vi "Index_Logic.vi"(0 "X":bool, 4 "Intake Pressed":bool, 6 "B":bool, 7 "Right Trigger":dbl, 8 "Y":bool, 9 "A":bool, 10 "Reject Pressed":bool, 11 "Elevate Pressed":bool) -> ()   [LabVIEW 2020]
uses:
  <vilib>/Rock Robotics/WPI/ThirdParty/Phoenix-LabVIEW/Motor Controller/Controls/CTRE_Phoenix_MotorControl_ControlMode.ctl
  <vilib>/Rock Robotics/WPI/Solenoid/WPI_SolenoidValue.ctl
  <vilib>/Rock Robotics/Network Tables/NT Read String.vi
  <vilib>/Rock Robotics/Network Tables/NT Write Boolean.vi
  <vilib>/Rock Robotics/Network Tables/NT Write Number.vi
  <vilib>/Rock Robotics/WPI/Solenoid/WPI_SolenoidSetEnum.vi
panel:
  in  "Intake want":dbl=0.75
  in  "Elevate want":dbl=-0.35
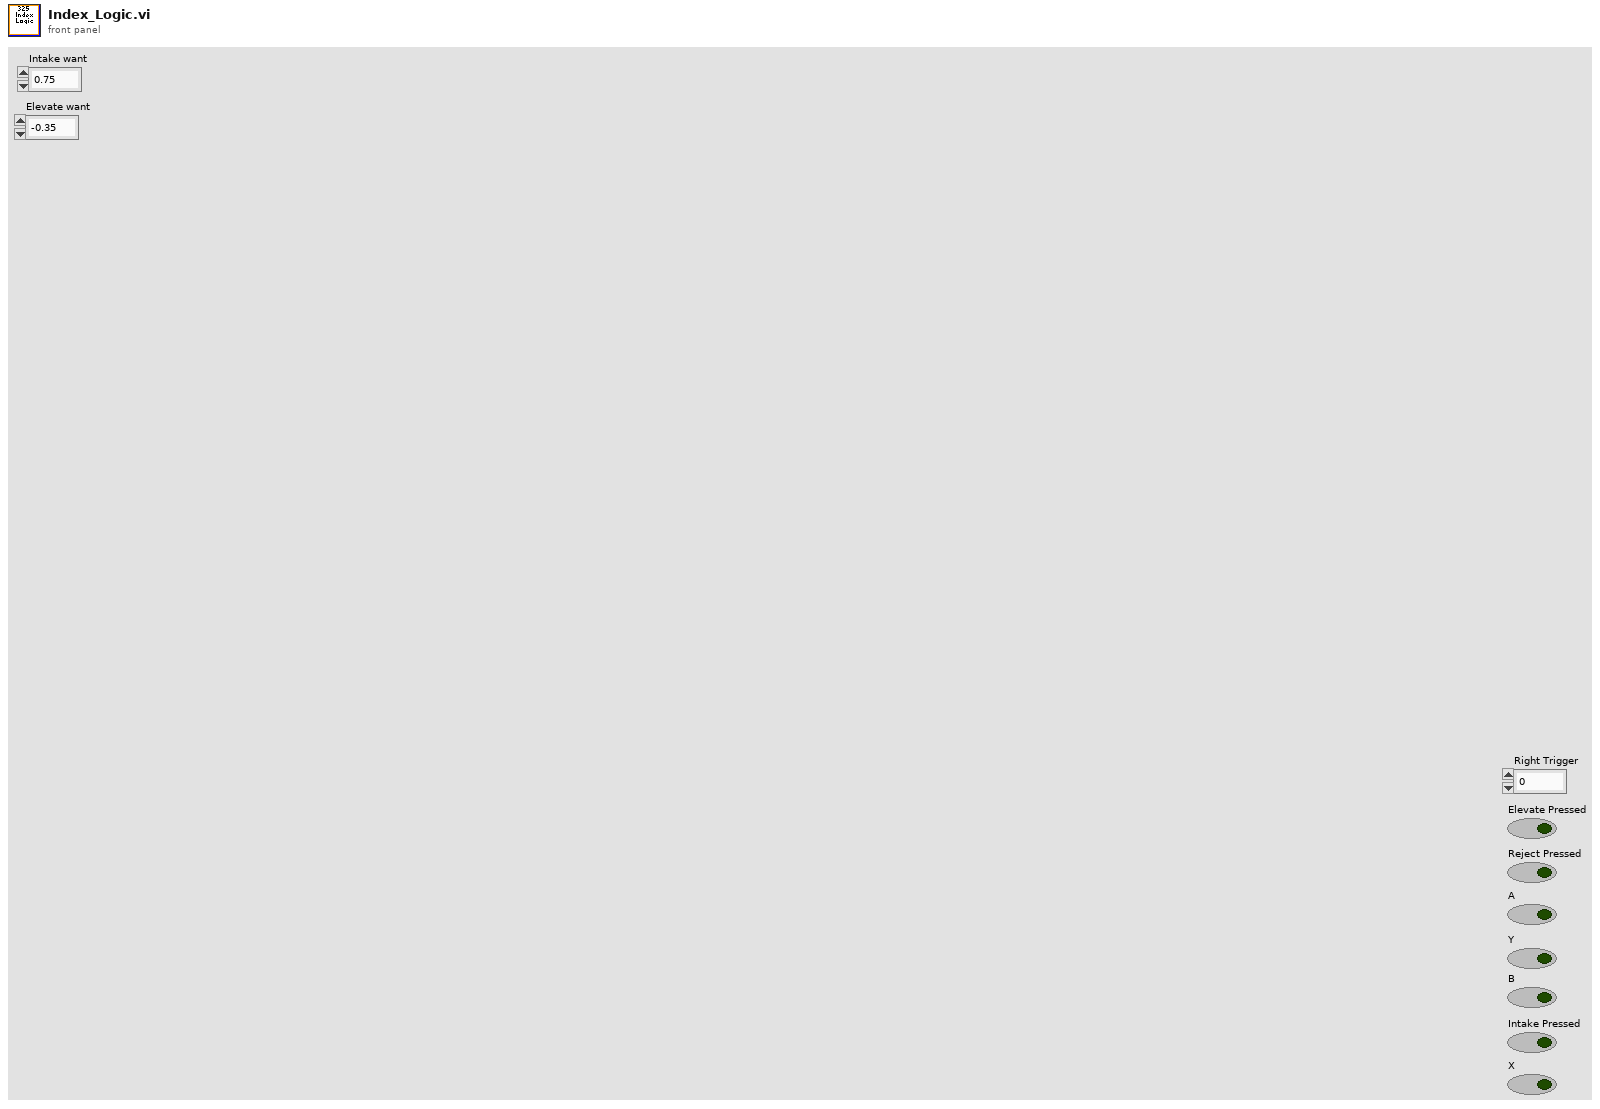
[diagram p1: front panel]
types:
  T1 = typedef "CTRE_Phoenix_MotorControl_ControlMode.ctl" = u16
  T2 = typedef "WPI_SolenoidValue.ctl" = enum16{"Off", "On", "Forward", "Reverse"}
  T3 = typedef "WPI_MotorControlDeviceRef.ctl" = cluster{"DeviceStatus":errorcluster, "Type":T4, "PWM":cluster{"PWM Channel":T5, "DeadBand":T6}, "CAN":cluster{"Device Number":u8, "SetOutput VI Ref":variant, "GetOutput VI Ref":variant, "Enable VI Ref":variant, "Disable VI Ref":variant, "Data":variant}, "Invert":bool, "DIO PWM":cluster{"PWM \"Enable\" Channel":T5, "DIOChannel":T7, "PWM Rate":dbl}}
  T4 = typedef "WPI_MotorControlType.ctl" = enum16{"PWM", "CAN", "DIO PWM"}
  T5 = typedef "FPGA_DIOPWMChannel.ctl" = enum8{"PWM 0", "PWM 1", "PWM 2", "PWM 3", "PWM 4", "PWM 5", "PWM 6", "PWM 7", "PWM 8", "PWM 9", "PWM MXP 0", "PWM MXP 1", "PWM MXP 2", "PWM MXP 3", "PWM MXP 4", "PWM MXP 5", "PWM MXP 6", "PWM MXP 7", "PWM MXP 8", "PWM MXP 9", "Invalid"}
  T6 = typedef "WPI_PWMDeadband.ctl" = cluster{"Name":string, "maxPositivePwm":i32, "minPositivePwm":i32, "centerPwm":i32, "maxNegativePwm":i32, "minNegativePwm":i32, "angularRange":u16}
  T7 = typedef "FPGA_DIOChannel.ctl" = enum8{"DIO 0", "DIO 1", "DIO 2", "DIO 3", "DIO 4", "DIO 5", "DIO 6", "DIO 7", "DIO 8", "DIO 9", "DIO MXP 0", "DIO MXP 1", "DIO MXP 2", "DIO MXP 3", "DIO MXP 4", "DIO MXP 5", "DIO MXP 6", "DIO MXP 7", "DIO MXP 8", "DIO MXP 9", "DIO MXP 10", "DIO MXP 11", "DIO MXP 12", "DIO MXP 13", "DIO MXP 14", "DIO MXP 15", "SPI Port CS1", "SPI Port CS2", "SPI Port CS3", "SPI Port MISO", "SPI Port MOSI", "Invalid"}
  T8 = typedef "WPI_SolenoidDevRef.ctl" = cluster{"DevStatus":errorcluster, "Pneumatics Control Module":u8, "Forward Solenoid Channel":T9, "Reverse Solenoid Channel":T9}
  T9 = typedef "WPI_SolenoidChannel.ctl" = enum8{"Solenoid 0", "Solenoid 1", "Solenoid 2", "Solenoid 3", "Solenoid 4", "Solenoid 5", "Solenoid 6", "Solenoid 7", "Solenoid 8", "Solenoid 9", "Solenoid 10", "Solenoid 11", "Solenoid 12", "Solenoid 13", "Solenoid 14", "Solenoid 15", "Invalid"}
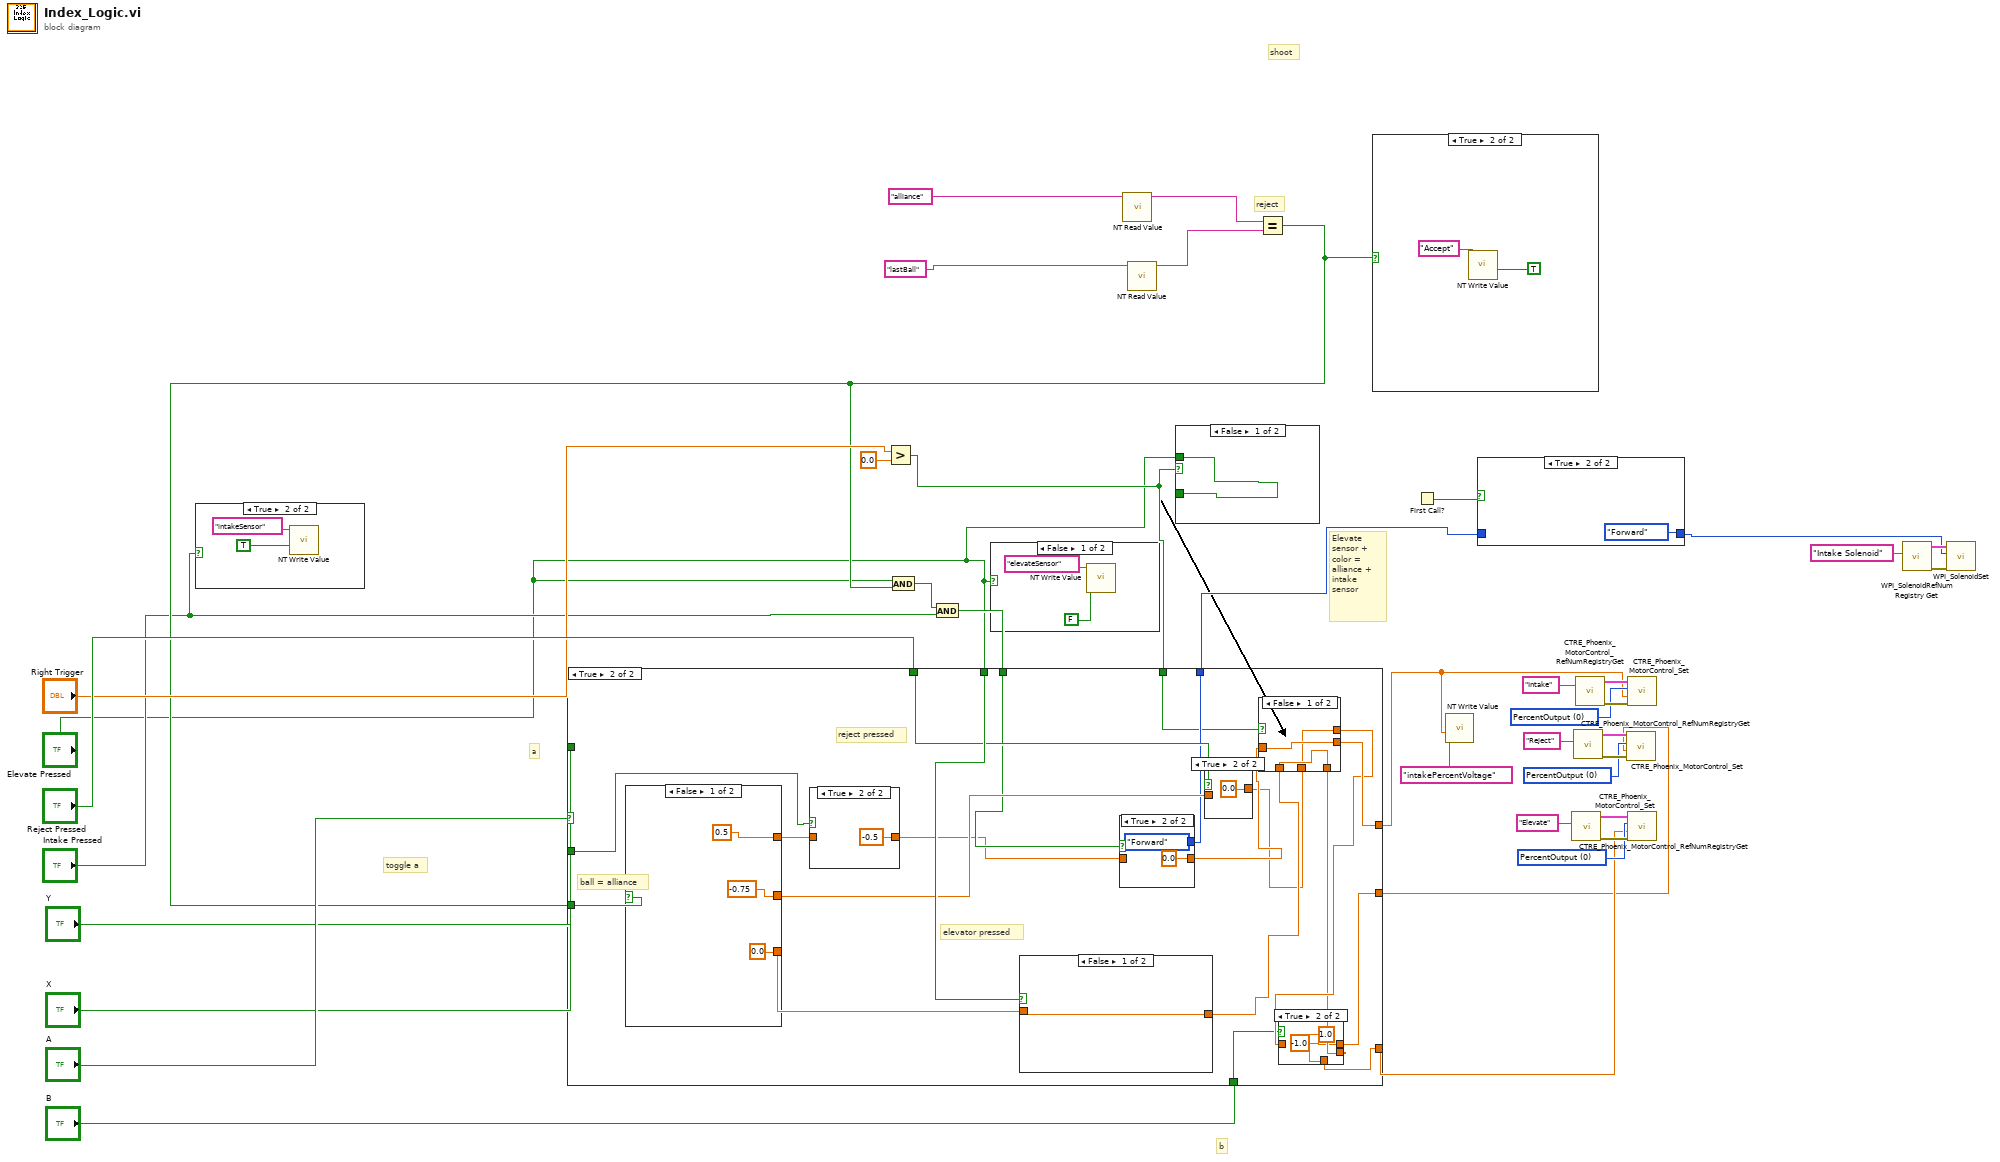
[diagram p0: block diagram]
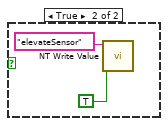
[diagram p3: hidden frame]
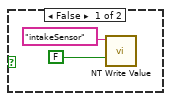
[diagram p4: hidden frame]
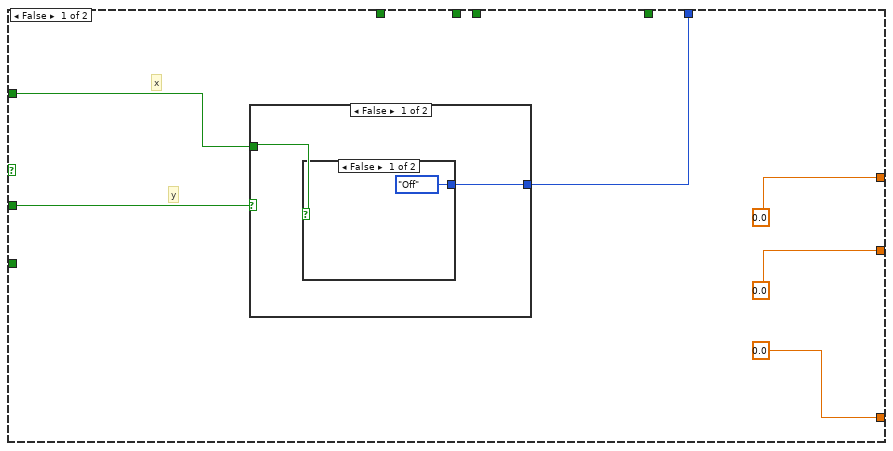
[diagram p5: hidden frame]
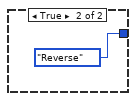
[diagram p6: hidden frame]
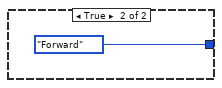
[diagram p7: hidden frame]
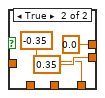
[diagram p10: hidden frame]
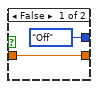
[diagram p11: hidden frame]
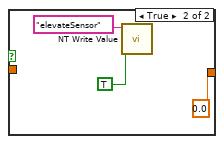
[diagram p13: hidden frame]
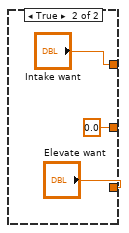
[diagram p14: hidden frame]
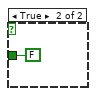
[diagram p15: hidden frame]
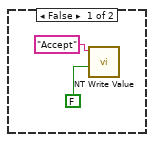
[diagram p16: hidden frame]
diagram:
  w28 = T1 0 items=["PercentOutput"=0, "Position"=1, "Velocity"=2, "Current"=3, "Follower"=5, "MotionProfile"=6, "MotionMagic"=7, "MotionProfileArc"=10, "Disabled"=15] ("Control Mode")
  w29 = T1 0 items=["PercentOutput"=0, "Position"=1, "Velocity"=2, "Current"=3, "Follower"=5, "MotionProfile"=6, "MotionMagic"=7, "MotionProfileArc"=10, "Disabled"=15] ("Control Mode")
  w30 = T1 0 items=["PercentOutput"=0, "Position"=1, "Velocity"=2, "Current"=3, "Follower"=5, "MotionProfile"=6, "MotionMagic"=7, "MotionProfileArc"=10, "Disabled"=15] ("Control Mode")
  # "toggle a"
  # "Elevate sensor + color = alliance + intake sensor"
  # "b"
  # "a"
  # "shoot"
  # "reject"
  n1 = case shown="True" "Intake Pressed" {
    frame False {
      n2 = call-poly <vilib>:"NT Write Value.vi"("Boolean"=FALSE, "Name"="intakeSensor") -> ()  [unwired: 9 in, 1 out]
    }
    frame True {
      n3 = call-poly <vilib>:"NT Write Value.vi"("Boolean"=TRUE, "Name"="intakeSensor") -> ()  [unwired: 9 in, 1 out]
    }
  }
  n4 = Greater?(x="Right Trigger", y=0.0) -> (0:w15:bool)
  n5 = case shown="False" "Elevate Pressed" {
    frame False {
      n6 = call-poly <vilib>:"NT Write Value.vi"("Boolean"=FALSE, "Name"="elevateSensor") -> ()  [unwired: 9 in, 1 out]
    }
    frame True {
      n7 = call-poly <vilib>:"NT Write Value.vi"("Boolean"=TRUE, "Name"="elevateSensor") -> ()  [unwired: 9 in, 1 out]
    }
  }
  n8 = call-poly <vilib>:"NT Read Value.vi"("Name"="alliance") -> ("String"=w27:string)  [unwired: 9 in, 1 out]
  n9 = call-poly <vilib>:"NT Read Value.vi"("Name"="lastBall") -> ("String"=w24:string)  [unwired: 9 in, 1 out]
  n10 = case shown="False" w15 {
    tunnel: "Elevate Pressed" -> [w48 _]
    tunnel: [w48 FALSE ("Switch Pressed")] -> _
    frame False {
    }
    frame True {
    }
  }
  n11 = Equal?(x=w27, y=w24) -> (x = y?=w8:bool)
  n12 = And(x="Elevate Pressed", y=w8) -> (x .and. y?=w18:bool)
  n13 = And(x=w18, y="Intake Pressed") -> (x .and. y?=w17:bool)
  n14 = case shown="True" "A" {
    tunnel: w8 -> [_ w80]
    tunnel: [0.0 ("Intake want") w73] -> w7
    tunnel: [0.0 ("Elevate 1") w65] -> w20
    tunnel: "Elevate Pressed" -> [_ w79]
    tunnel: [0.0 ("Reject no want") w68] -> w19
    tunnel: "Reject Pressed" -> [_ w77]
    tunnel: w17 -> [_ w64]
    tunnel: [w52 w75] -> w3
    tunnel: w15 -> [_ w71]
    tunnel: "B" -> [_ w67]
    tunnel: "Y" -> [w51 w63]
    tunnel: "X" -> [w50 _]
    frame False {
      # "x"
      # "y"
      n15 = case shown="False" w51 {
        tunnel: [w57 WPI_SolenoidValue."Forward" ("Value")] -> w52
        tunnel: w50 -> [w56 _]
        frame False {
          n16 = case shown="False" w56 {
            tunnel: [WPI_SolenoidValue."Off" ("Value") WPI_SolenoidValue."Reverse" ("Value")] -> w57
            frame False {
            }
            frame True {
            }
          }
        }
        frame True {
        }
      }
    }
    frame True {
      # "reject pressed"
      # "elevator pressed"
      # "ball = alliance"
      n17 = case shown="False" w80 {
        tunnel: [0.0 ("Elevate want") "Elevate want"] -> w78
        tunnel: [0.5 ("Intake 1") "Intake want"] -> w61
        tunnel: [-0.75 ("Reject no want") 0.0 ("Reject no want")] -> w76
        frame False {
        }
        frame True {
        }
      }
      n18 = case shown="True" w63 {
        tunnel: [w81 -0.5 ("Intake want")] -> w62
        tunnel: w61 -> [w81 _]
        frame False {
        }
        frame True {
        }
      }
      n19 = case shown="False" w79 {
        tunnel: [w99 0.0 ("Elevate 1")] -> w72
        tunnel: w78 -> [w99 _]
        frame False {
        }
        frame True {
          n20 = call-poly <vilib>:"NT Write Value.vi"("Boolean"=TRUE, "Name"="elevateSensor") -> ()  [unwired: 9 in, 1 out]
        }
      }
      n21 = case shown="True" w64 {
        tunnel: w62 -> [w94 _]
        tunnel: [w94 0.0 ("Intake want")] -> w74
        tunnel: [WPI_SolenoidValue."Off" ("Value") WPI_SolenoidValue."Forward" ("Value")] -> w75
        frame False {
        }
        frame True {
        }
      }
      n22 = case shown="True" w77 {
        tunnel: w76 -> [w97 _]
        tunnel: [w97 0.0 ("Reject no want")] -> w70
        frame False {
        }
        frame True {
        }
      }
      n23 = case shown="False" w71 {
        tunnel: w74 -> [w89 _]
        tunnel: [w89 0.35 ("Intake want")] -> w73
        tunnel: w72 -> [w88 _]
        tunnel: [w88 -0.35 ("Elevate 1")] -> w66
        tunnel: w70 -> [w87 _]
        tunnel: [w87 0.0 ("Reject no want")] -> w69
        frame False {
        }
        frame True {
        }
      }
      n24 = case shown="True" w67 {
        tunnel: w69 -> [w84 _]
        tunnel: [w84 -1.0 ("Reject no want")] -> w68
        tunnel: w66 -> [w83 _]
        tunnel: [w83 1.0 ("Elevate 1")] -> w65
        frame False {
        }
        frame True {
        }
      }
    }
  }
  n25 = case shown="True" w8 {
    frame False {
      n26 = call-poly <vilib>:"NT Write Value.vi"("Boolean"=FALSE, "Name"="Accept") -> ()  [unwired: 9 in, 1 out]
    }
    frame True {
      n27 = call-poly <vilib>:"NT Write Value.vi"("Boolean"=TRUE, "Name"="Accept") -> ()  [unwired: 9 in, 1 out]
    }
  }
  n28 = First Call?() -> (First Call?: T/F=w1:bool)
  n29 = call-poly <vilib>:"NT Write Value.vi"("Numeric"=w7, "Name"="intakePercentVoltage") -> ()  [unwired: 9 in, 1 out]
  n30 = case shown="True" w1 {
    tunnel: w3 -> [w113 _]
    tunnel: [w113 WPI_SolenoidValue."Forward" ("Value")] -> w2
    frame False {
    }
    frame True {
    }
  }
  n31 = call <vilib>:"CTRE_Phoenix_MotorControl_RefNumRegistryGet.vi"("refnum name"="Elevate") -> ("error out"=w35:errorcluster, "PhoenixMotorControlDevRef"=w34:T3)  [unwired: 9 in]
  n32 = call <vilib>:"CTRE_Phoenix_MotorControl_RefNumRegistryGet.vi"("refnum name"="Reject") -> ("error out"=w37:errorcluster, "PhoenixMotorControlDevRef"=w36:T3)  [unwired: 9 in]
  n33 = call <vilib>:"CTRE_Phoenix_MotorControl_RefNumRegistryGet.vi"("refnum name"="Intake") -> ("error out"=w39:errorcluster, "PhoenixMotorControlDevRef"=w38:T3)  [unwired: 9 in]
  n34 = call <vilib>:"CTRE_Phoenix_MotorControl_Set.vi"("error in (no error)"=w37, "Output"=w19, "Control Mode"=w28, "PhoenixMotorControlDevRef"=w36) -> ()  [unwired: 6 in, 2 out]
  n35 = call <vilib>:"CTRE_Phoenix_MotorControl_Set.vi"("error in (no error)"=w39, "Output"=w7, "Control Mode"=w29, "PhoenixMotorControlDevRef"=w38) -> ()  [unwired: 6 in, 2 out]
  n36 = call <vilib>:"CTRE_Phoenix_MotorControl_Set.vi"("error in (no error)"=w35, "Output"=w20, "Control Mode"=w30, "PhoenixMotorControlDevRef"=w34) -> ()  [unwired: 6 in, 2 out]
  n37 = call <vilib>:"WPI_SolenoidRefNum Registry Get.vi"("refnum name"="Intake Solenoid") -> ("error out"=w23:errorcluster, "SolenoidDevRef"=w22:T8)  [unwired: 9 in]
  n38 = call-poly <vilib>:"WPI_SolenoidSet.vi"("error in (no error)"=w23, "Value"=w2, "SolenoidDevRef"=w22) -> ()  [unwired: 7 in, 2 out]
